vi "校准任务设置.vi"(11 "用户事件":refnum<user-event>) -> ()   [LabVIEW 2016, in "斯坦道CODMn新电路板.lvlib"]
panel:
  in  "校准任务存档":T1[](array[typedef])
  out "字符串":string
  out "校准运行状态":bool
  in  "校准任务":T1[](array[typedef])
  in  "停止":bool
  in  "设置":bool
  in  "执行":bool
  in  "删除":bool
  in  "清空":bool
  in  "任务列表":i32(listbox)
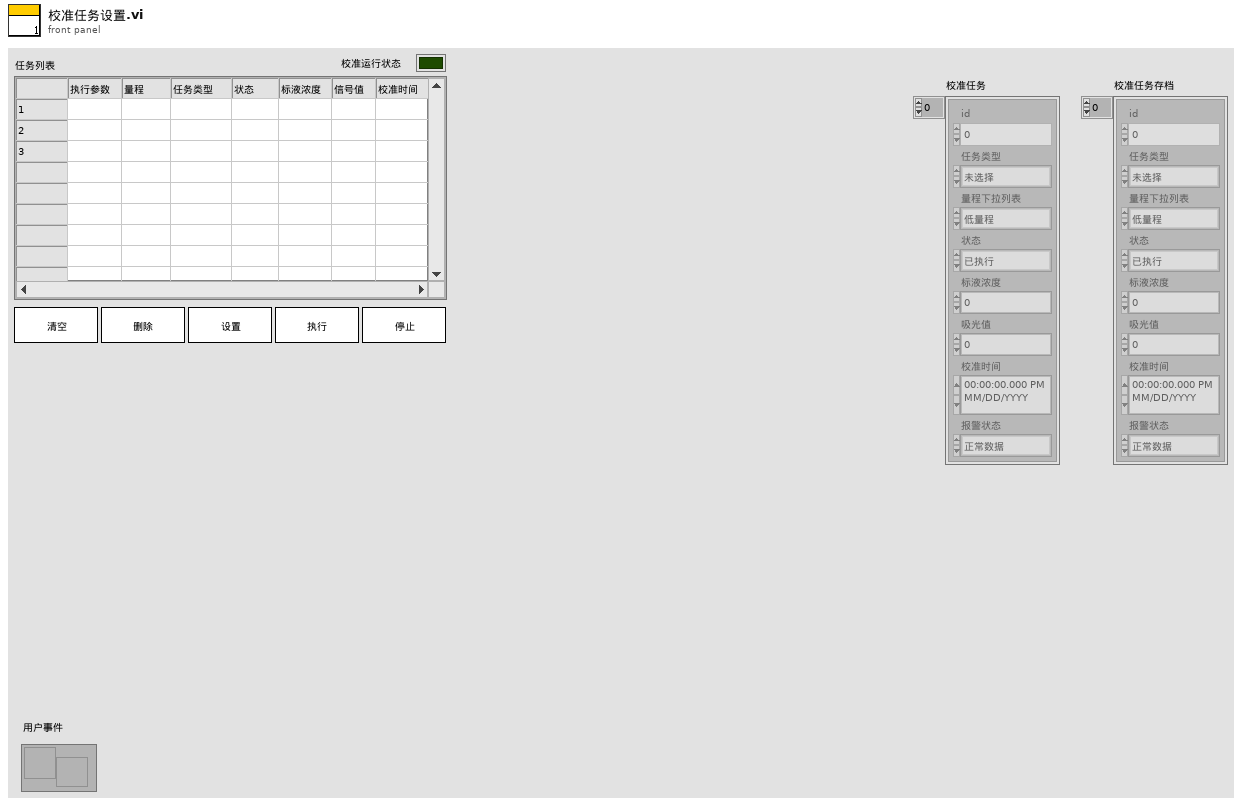
[diagram p1: front panel]
types:
  T1 = typedef "校准任务.ctl" = cluster{"id":u16, "任务类型":enum16{"未选择", "空白校准", "标样校准", "标样核查", "零点核查", "跨度核查"}, "量程下拉列表":enum16{"低量程", "高量程"}, "状态":enum16{"已执行", "待执行", "执行中", "停止"}, "标液浓度":dbl, "吸光值":dbl, "校准时间":timestamp, "报警状态":enum16{"正常数据", "报警数据"}}
  T2 = cluster{"校准类型":string, "校准数据":cluster{"时间":timestamp, "标液值":dbl, "检测值":dbl, "吸光值":dbl}}
  T3 = enum8{"Enabled", "Disabled", "Disabled and Grayed Out"}
  T4 = typedef "LVPoint32TypeDef.ctl" = cluster{"Horizontal":i32, "Vertical":i32}
  T5 = typedef "LVRowAndColumnTypeDef.ctl" = cluster{"Row":i32, "Column":i32}
  T6 = enum16{"未选择", "空白校准", "标样校准", "标样核查", "零点核查", "跨度核查"}
  T7 = cluster{"id":u16, "任务类型":enum16{"未选择", "空白校准", "标样校准", "标样核查", "零点核查", "跨度核查"}, "量程下拉列表":enum16{"低量程", "高量程"}, "状态":enum16{"已执行", "待执行", "执行中", "停止"}, "标液浓度":dbl, "吸光值":dbl, "校准时间":timestamp, "报警状态":enum16{"正常数据", "报警数据"}}
  T8 = enum32{"Bad", "Idle", "Run top level", "Running"}
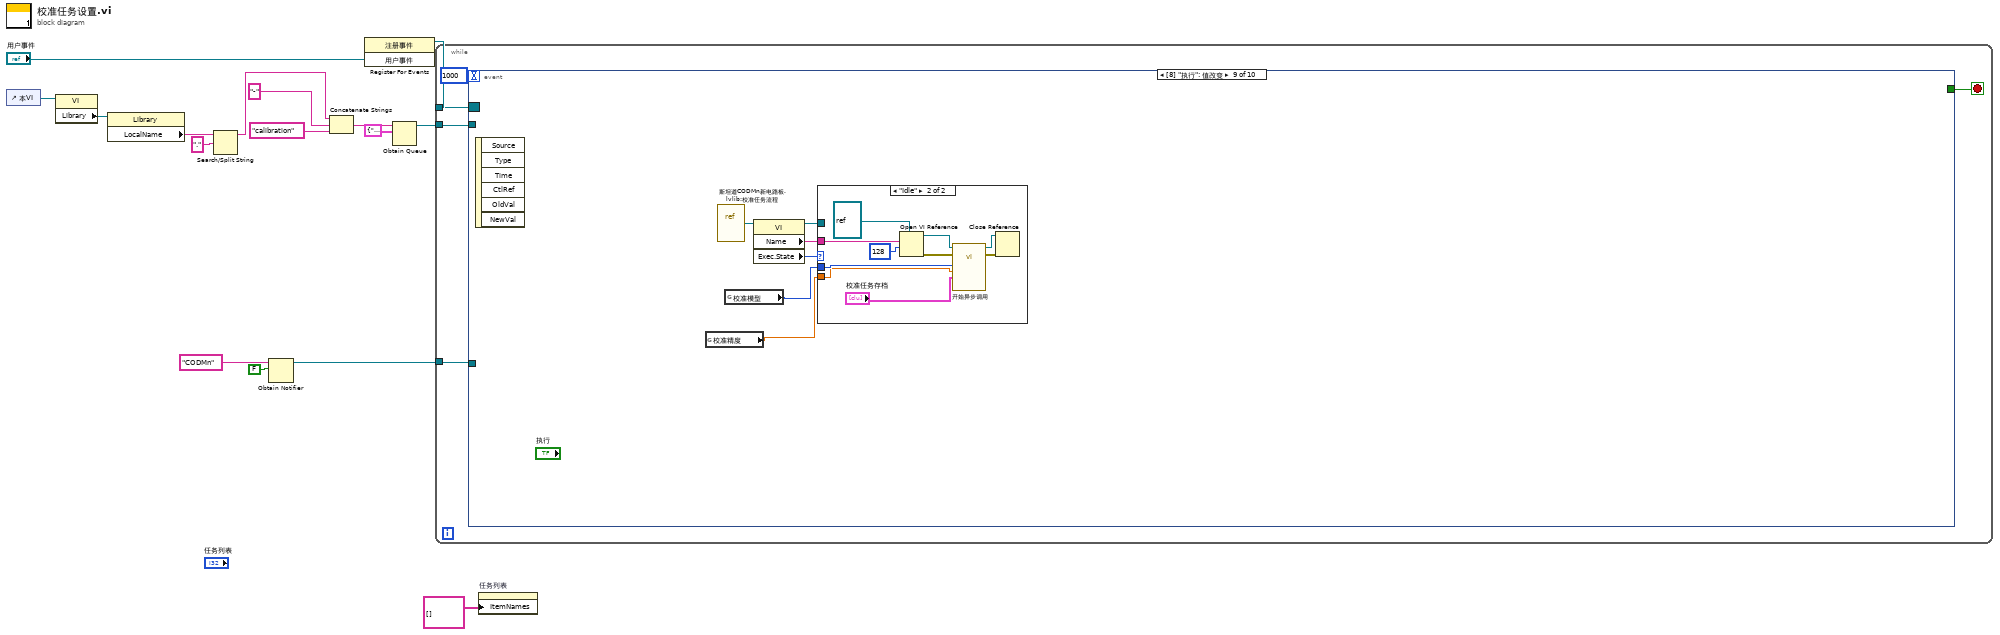
[diagram p0: block diagram]
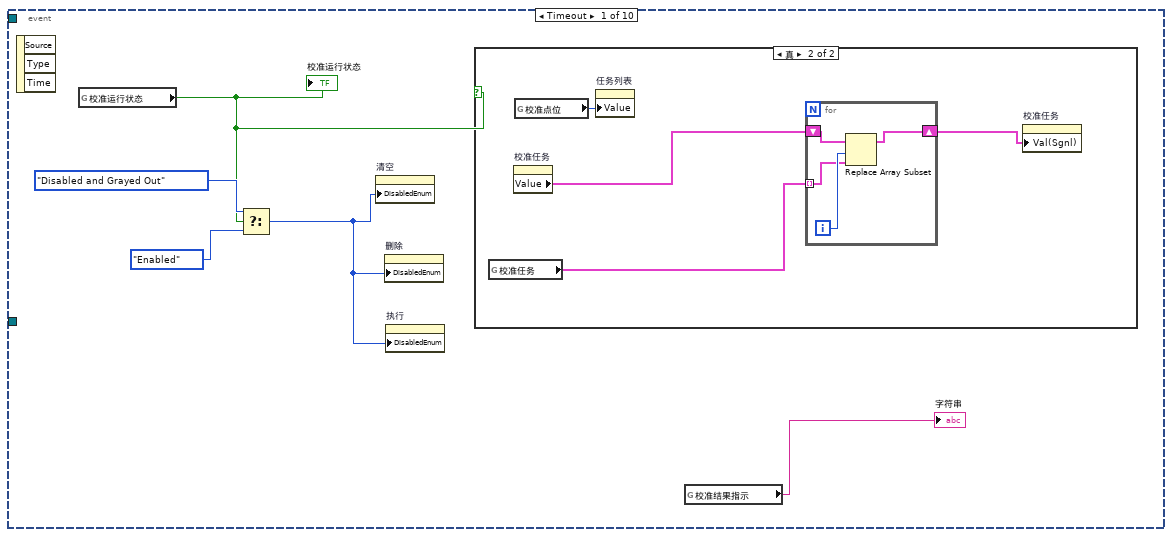
[diagram p2: hidden frame]
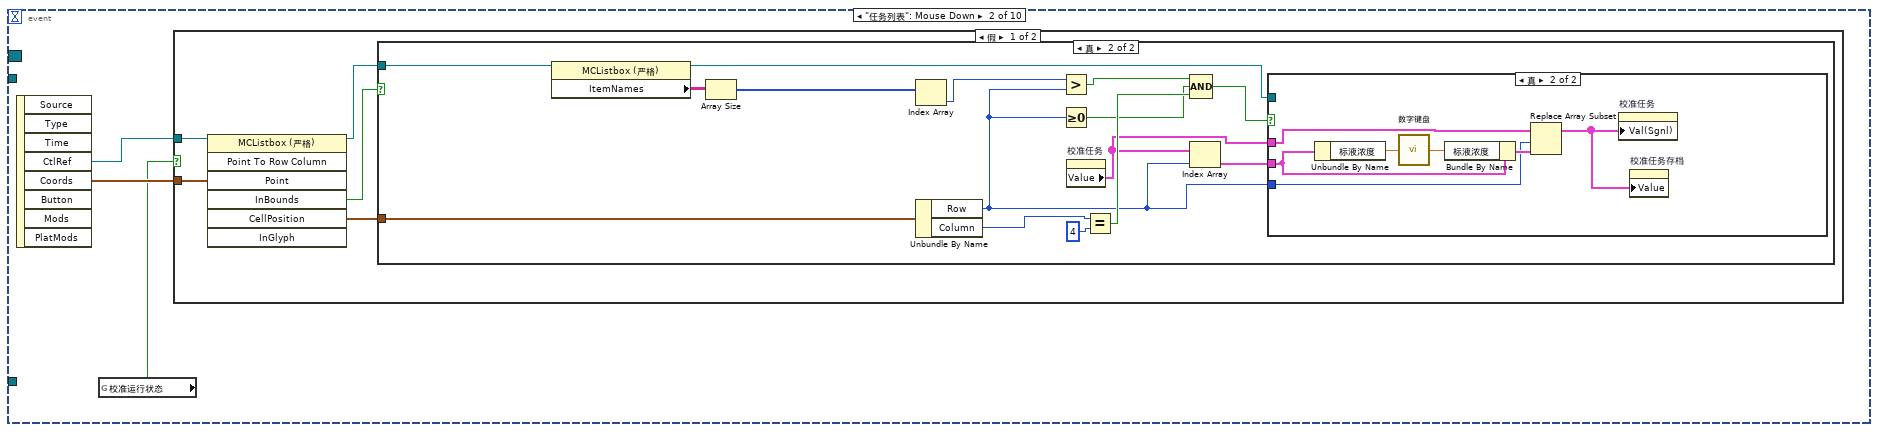
[diagram p4: hidden frame]
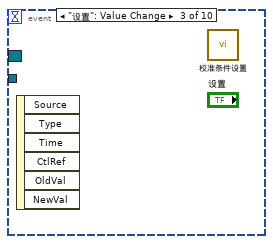
[diagram p8: hidden frame]
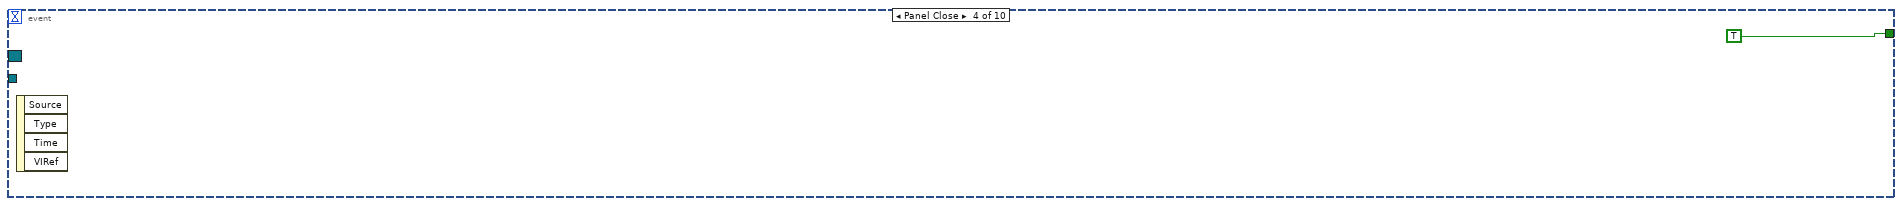
[diagram p9: hidden frame]
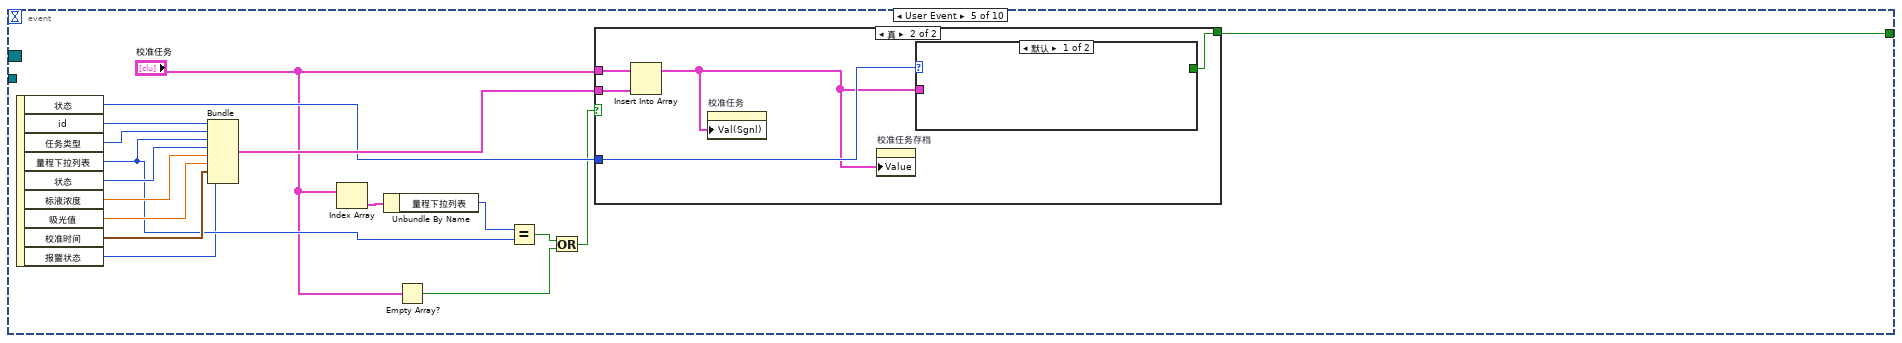
[diagram p10: hidden frame]
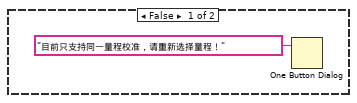
[diagram p11: hidden frame]
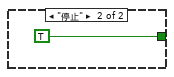
[diagram p12: hidden frame]
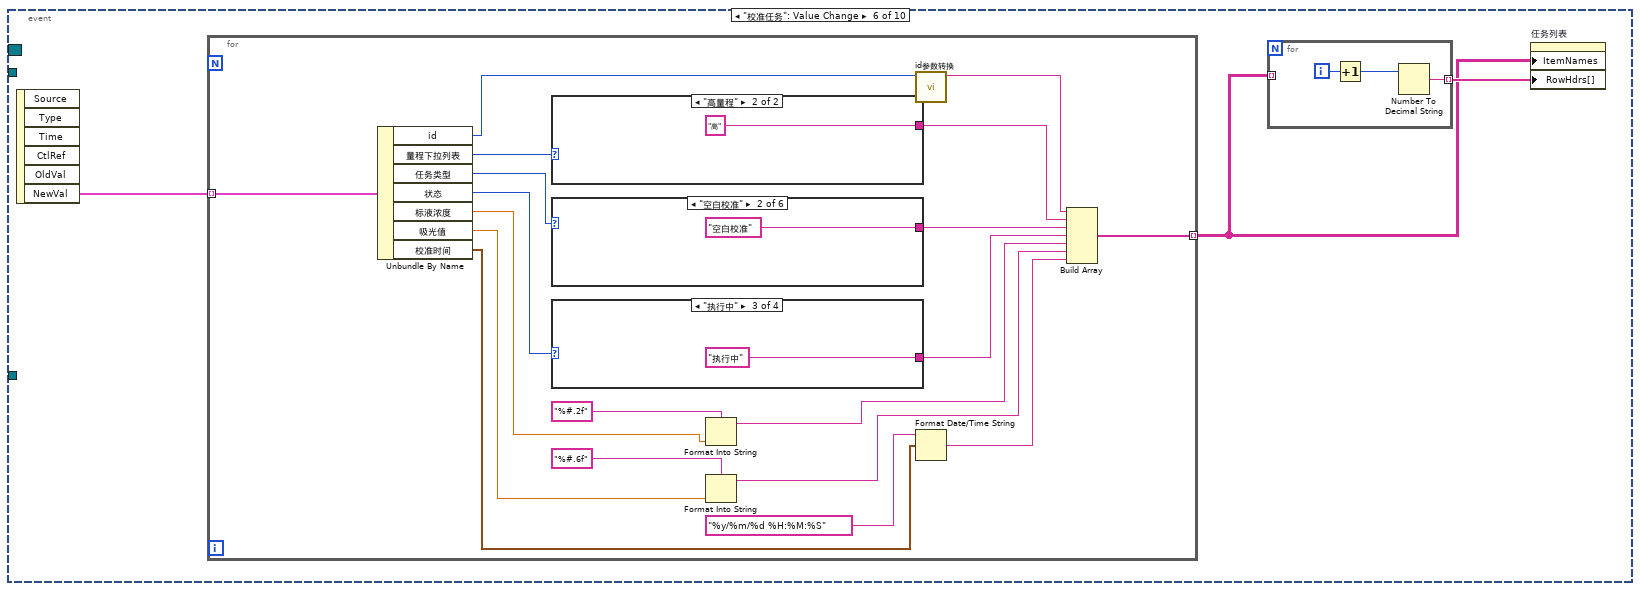
[diagram p13: hidden frame]
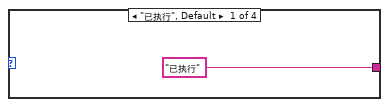
[diagram p14: hidden frame]
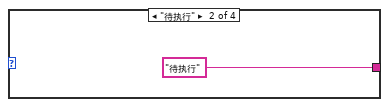
[diagram p15: hidden frame]
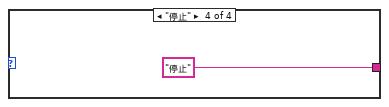
[diagram p16: hidden frame]
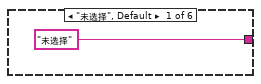
[diagram p17: hidden frame]
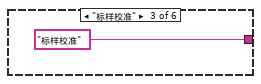
[diagram p18: hidden frame]
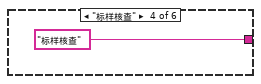
[diagram p19: hidden frame]
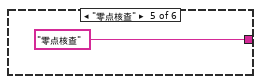
[diagram p20: hidden frame]
diagram:
  n1 = control-ref of="本VI"() -> (w15:refnum<vi>)
  n2 = property class="VI"(reference=w15) -> ("Library"=w16:refnum<vi>)  [unwired: 1 in, 2 out]
  n3 = property class="Library"(reference=w16) -> ("LocalName"=w14:string)  [unwired: 1 in, 2 out]
  n4 = Search/Split String(string=w14, search string/char (-)="." ("搜索字符串/字符(-)")) -> (substring before match=w12:string)  [unwired: 1 in, 2 out]
  n5 = Obtain Notifier(name (unnamed)="CODMn" ("字符串"), notification data type=FALSE) -> (notifier out=w3:refnum<notifier>)  [unwired: 2 in, 2 out]
  n6 = Concatenate Strings(w12, "-" ("字符串"), "calibration" ("名称或相对路径")) -> (w9:string)
  n7 = register-events("用户事件") -> (reference out=w6:refnum<event-registration>)  [unwired: 2 in, 1 out]
  n8 = Obtain Queue(name (unnamed)=w9, element data type=T2 {"校准类型"="", "校准数据"={"时间"=timestamp(0 s since 1904-01-01), "标液值"=0.0, "检测值"=0.0, "吸光值"=0.0}}) -> (queue out=w7:refnum<queue>)  [unwired: 3 in, 2 out]
  n9 = while {
    tunnel: w7 -> [w20]
    tunnel: w6 -> [w19]
    tunnel: w3 -> [w18]
    stop <- w21 stop-if-true
    n10 = event shown="[8] \"执行\": 值改变" {
      selector: w19 -> [_ _ _ _ _ _ _ _ _ _]
      dyn-events: _ -> [_ _ _ _ _ _ _ _ _ _]
      timeout: 1000 -> [_ _ _ _ _ _ _ _ _ _]
      tunnel: [_ _ _ TRUE w82 _ _ _ _ _] -> w21
      tunnel: w20 -> [_ _ _ _ _ _ _ _ _ _]
      tunnel: w18 -> [_ _ _ _ _ _ _ _ _ w148]
      event Timeout {
        n11 = event-data() -> ()  [unwired: 1 in, 3 out]
        n12 = global read "VARCODMn全局变量.vi" "校准运行状态"() -> (w23:bool)
        "校准运行状态" <- w23
        n13 = Select(t=T3."Disabled and Grayed Out" ("禁用"), s=w23, f=T3."Enabled" ("禁用")) -> (s? t:f=w25:T3)
        n14 = property on="清空" class="Bool"("DisabledEnum"=w25) -> ()  [unwired: 2 in, 2 out]
        n15 = property on="删除" class="Bool"("DisabledEnum"=w25) -> ()  [unwired: 2 in, 2 out]
        n16 = property on="执行" class="Bool"("DisabledEnum"=w25) -> ()  [unwired: 2 in, 2 out]
        n17 = case shown="真" w23 {
          frame False {
          }
          frame True {
            n18 = global read "VARCODMn全局变量.vi" "校准任务"() -> (w28:T1[])
            n19 = property on="校准任务" class="Arr (严格)"() -> ("Value"=w29:T1[])  [unwired: 2 in, 2 out]
            n20 = global read "VARCODMn全局变量.vi" "校准点位"() -> (w30:u16)
            n21 = property on="任务列表" class="MCListbox (严格)"("Value"=w30) -> ()  [unwired: 2 in, 2 out]
            n22 = for {
              tunnel: w28 -> [w32] mode=indexing
              shift-right: [w31] -> w27
              shift-left: w29 -> [w34]
              i -> [w33]
              n23 = Replace Array Subset(array=w34, new element=w32, index=w33) -> (w31:T1[])
            }
            n24 = property on="校准任务" class="Arr (严格)"("Val(Sgnl)"=w27) -> ()  [unwired: 2 in, 2 out]
          }
        }
        n25 = global read "VARCODMn全局变量.vi" "校准结果指示"() -> (→"字符串":string)
      }
      event "任务列表": Mouse Down {
        n26 = event-data() -> ("CtlRef"=w37:refnum<vi>, "Coords"=w36:T4)  [unwired: 1 in, 6 out]
        n27 = global read "VARCODMn全局变量.vi" "校准运行状态"() -> (w35:bool)
        n28 = case shown="假" w35 {
          tunnel: w37 -> [w42 _]
          tunnel: w36 -> [w38 _]
          frame False {
            n29 = invoke class="MCListbox (严格)" method="Point To Row Column"(reference=w42, "Point"=w38) -> (reference out=w39:refnum<vi>, "InBounds"=w41:bool, "CellPosition"=w40:T5)  [unwired: 5 in, 4 out]
            n30 = case shown="真" w41 {
              tunnel: w40 -> [_ w57]
              tunnel: w39 -> [_ w56]
              frame False {
              }
              frame True {
                n31 = property class="MCListbox (严格)"(reference=w56) -> (reference out=w55:refnum<vi>, "ItemNames"=w54:string[][])  [unwired: 1 in, 1 out]
                n32 = Array Size(array=w54) -> (size(s)=w53:i32[])
                n33 = Index Array(array=w53) -> (element=w52:i32)  [unwired: 1 in]
                n34 = Unbundle By Name(w57) -> ("Row"=w43:i32, "Column"=w51:i32)
                n35 = Greater?(x=w52, y=w43) -> (0:w47:bool)
                n36 = Greater Or Equal To 0?(x=w43) -> (x >= 0?=w46:bool)
                n37 = property on="校准任务" class="Arr (严格)"() -> ("Value"=w44:T1[])  [unwired: 2 in, 2 out]
                n38 = Equal?(x=w51, y=4) -> (x = y?=w49:bool)
                n39 = Compound Arithmetic op=AND ("复合运算")(w47, w46, w49) -> (w48:bool)
                n40 = Index Array(array=w44, index=w43) -> (element=w45:T1)
                n41 = case shown="真" w48 {
                  tunnel: w55 -> [_ _]
                  tunnel: w45 -> [_ w63]
                  tunnel: w44 -> [_ w61]
                  tunnel: w43 -> [_ w59]
                  frame False {
                  }
                  frame True {
                    n42 = Unbundle By Name(w63) -> ("标液浓度"=w64:dbl)
                    n43 = call "数字键盘.vi"("OldNumber"=w64) -> ("NewNumber"=w62:dbl)
                    n44 = Bundle By Name(cluster=w63, "标液浓度"=w62) -> (w60:T1)
                    n45 = Replace Array Subset(array=w61, new element=w60, index=w59) -> (w58:T1[])
                    n46 = property on="校准任务" class="Arr (严格)"("Val(Sgnl)"=w58) -> ()  [unwired: 2 in, 2 out]
                    n47 = property on="校准任务存档" class="Arr (严格)"("Value"=w58) -> ()  [unwired: 2 in, 2 out]
                  }
                }
              }
            }
          }
          frame True {
          }
        }
      }
      event "设置": Value Change {
        n48 = event-data() -> ()  [unwired: 1 in, 6 out]
        n49 = call "校准条件设置.vi"() -> ()  [unwired: 12 in]
      }
      event Panel Close {
        n50 = event-data() -> ()  [unwired: 1 in, 4 out]
      }
      event User Event {
        n51 = event-data() -> ("状态"=w74:enum16{"已执行", "待执行", "执行中", "停止"}, "id"=w81:u16, "任务类型"=w79:T6, "量程下拉列表"=w71:enum16{"低量程", "高量程"}, "状态"=w78:enum16{"已执行", "待执行", "执行中", "停止"}, "标液浓度"=w77:dbl, "吸光值"=w76:dbl, "校准时间"=w75:timestamp, "报警状态"=w66:enum16{"正常数据", "报警数据"})  [unwired: 1 in]
        n52 = Bundle("id"=w81, "任务类型"=w79, "量程下拉列表"=w71, "状态"=w78, "标液浓度"=w77, "吸光值"=w76, "校准时间"=w75, "报警状态"=w66) -> (w80:T7)  [unwired: 1 in]
        n53 = Index Array(array="校准任务") -> (element=w73:T1)  [unwired: 1 in]
        n54 = Unbundle By Name(w73) -> ("量程下拉列表"=w72:enum16{"低量程", "高量程"})
        n55 = Empty Array?(array="校准任务") -> (empty?=w67:bool)
        n56 = Equal?(x=w72, y=w71) -> (x = y?=w69:bool)
        n57 = Or(x=w69, y=w67) -> (x .or. y?=w68:bool)
        n58 = case shown="真" w68 {
          tunnel: [_ w88] -> w82
          tunnel: w80 -> [_ w87]
          tunnel: w74 -> [_ w86]
          tunnel: "校准任务" -> [_ w85]
          frame False {
            n59 = One Button Dialog(message="目前只支持同一量程校准，请重新选择量程！" ("消息")) -> ()  [unwired: 1 in, 1 out]
          }
          frame True {
            n60 = Insert Into Array(array=w85, new element=w87) -> (w84:T1[])  [unwired: 1 in]
            n61 = property on="校准任务" class="Arr (严格)"("Val(Sgnl)"=w84) -> ()  [unwired: 2 in, 2 out]
            n62 = property on="校准任务存档" class="Arr (严格)"("Value"=w84) -> ()  [unwired: 2 in, 2 out]
            n63 = case shown="默认" w86 {
              tunnel: [_ TRUE] -> w88
              tunnel: w84 -> [_ _]
              frame Default {
              }
              frame "停止" {
              }
            }
          }
        }
      }
      event "校准任务": Value Change {
        n64 = event-data() -> ("NewVal"=w90:T1[])  [unwired: 1 in, 5 out]
        n65 = for {
          tunnel: w90 -> [w111] mode=indexing
          tunnel: [w93] -> w91 mode=indexing
          n66 = Unbundle By Name(w111) -> ("id"=w110:u16, "量程下拉列表"=w109:enum16{"低量程", "高量程"}, "任务类型"=w108:T6, "状态"=w107:enum16{"已执行", "待执行", "执行中", "停止"}, "标液浓度"=w105:dbl, "吸光值"=w103:dbl, "校准时间"=w101:timestamp)
          n67 = case shown="\"高量程\"" w109 {
            tunnel: ["低" "高"] -> w99
            frame "低量程", Default {
            }
            frame "高量程" {
            }
          }
          n68 = case shown="\"空白校准\"" w108 {
            tunnel: ["未选择" "空白校准" "标样校准" "标样核查" "零点核查" "跨度核查"] -> w98
            frame "未选择", Default {
            }
            frame "空白校准" {
            }
            frame "标样校准" {
            }
            frame "标样核查" {
            }
            frame "零点核查" {
            }
            frame "跨度核查" {
            }
          }
          n69 = case shown="\"执行中\"" w107 {
            tunnel: ["已执行" "待执行" "执行中" "停止"] -> w97
            frame "已执行", Default {
            }
            frame "待执行" {
            }
            frame "执行中" {
            }
            frame "停止" {
            }
          }
          n70 = Format Into String(format string="%#.2f" ("格式字符串"), w105) -> (resulting string=w96:string)  [unwired: 2 in, 1 out]
          n71 = Format Into String(format string="%#.6f" ("格式字符串"), w103) -> (resulting string=w95:string)  [unwired: 2 in, 1 out]
          n72 = call "id参数转换.vi"("id"=w110) -> ("table输出"=w100:string)  [unwired: 10 in]
          n73 = Format Date/Time String(time format string (%c)="%y/%m/%d %H:%M:%S" ("时间格式字符串(%c)"), seconds (now)=w101) -> (date/time string=w94:string)  [unwired: 1 in]
          n74 = Build Array(w100, w99, w98, w97, w96, w95, w94) -> (w93:string[])
        }
        n75 = for {
          tunnel: [w124] -> w92 mode=indexing
          tunnel: w91 -> [_] mode=indexing
          i -> [w126]
          n76 = Increment(x=w126) -> (x+1=w125:i32)
          n77 = Number To Decimal String(number=w125) -> (decimal integer string=w124:string)  [unwired: 1 in]
        }
        n78 = property on="任务列表" class="MCListbox (严格)"("ItemNames"=w91, "RowHdrs[]"=w92) -> ()  [unwired: 2 in, 2 out]
      }
      event "清空": Value Change {
        n79 = event-data() -> ()  [unwired: 1 in, 6 out]
        n80 = property on="校准任务" class="Arr (严格)"("Val(Sgnl)"=T1[] [] ("数组")) -> ()  [unwired: 2 in, 2 out]
      }
      event "删除": Value Change {
        n81 = event-data() -> ()  [unwired: 1 in, 6 out]
        n82 = property on="校准任务" class="Arr (严格)"() -> ("Value"=w130:T1[])  [unwired: 2 in, 2 out]
        n83 = property on="任务列表" class="MCListbox (严格)"() -> ("Value"=w128:i32)  [unwired: 2 in, 2 out]
        n84 = Delete From Array(array=w130, index=w128) -> (array with subset deleted=w129:T1[])  [unwired: 1 in, 1 out]
        n85 = property on="校准任务" class="Arr (严格)"("Val(Sgnl)"=w129) -> ()  [unwired: 2 in, 2 out]
      }
      event "执行": Value Change {
        n86 = event-data() -> ()  [unwired: 1 in, 6 out]
        n87 = global read "VARCODMn全局变量.vi" "校准精度"() -> (w131:dbl)
        n88 = vi-ref "斯坦道CODMn新电路板.lvlib:校准任务流程.vi"() -> (w133:refnum<vi>)
        n89 = global read "VARCODMn全局变量.vi" "校准模型"() -> (w132:enum32{"线性", "多项式", "折线"})
        n90 = property class="VI"(reference=w133) -> (reference out=w136:refnum<vi>, "Name"=w134:string, "Exec.State"=w135:T8)  [unwired: 1 in, 1 out]
        n91 = case shown="\"Idle\"" w135 {
          tunnel: w134 -> [_ w146]
          tunnel: w136 -> [_ _]
          tunnel: w132 -> [_ w139]
          tunnel: w131 -> [_ w138]
          frame "Bad", Default {
          }
          frame "Idle" {
            n92 = Open VI Reference(type specifier VI Refnum (for type only)=refnum<vi> refnum, vi path=w146, options=128 ("选项")) -> (vi reference=w144:refnum<vi>, error out=w142:errorcluster)  [unwired: 3 in]
            n93 = call-by-ref "开始异步调用"(reference=w144, error in=w142, "校准任务"="校准任务存档", "精度"=w138, "模型"=w139) -> (reference out=w143:refnum<vi>, error out=w141:errorcluster)  [unwired: 9 in]
            n94 = Close Reference(reference=w143, error in (no error)=w141) -> ()  [unwired: 1 out]
          }
        }
      }
      event "停止": Value Change {
        n95 = event-data() -> ()  [unwired: 1 in, 6 out]
        n96 = Send Notification(notification=TRUE ("通知"), notifier=w148) -> ()  [unwired: 1 in, 2 out]
      }
    }
  }
  n97 = property on="任务列表" class="MCListbox (严格)"("ItemNames"=string[][] [] ("项名")) -> ()  [unwired: 2 in, 2 out]
